vi "Assert Test SubVI.vi"(8 "error in (no error)":errorcluster) -> (0 "error out":errorcluster)   [LabVIEW 2009]
uses:
  classes/Assert/Assert.lvclass
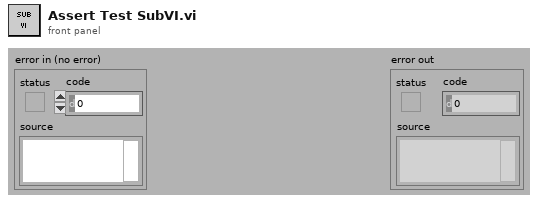
[diagram p1: front panel]
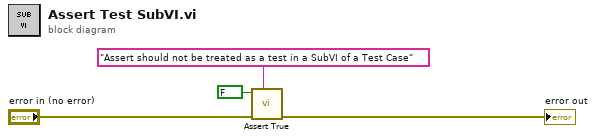
[diagram p0: block diagram]
diagram:
  n1 = call "Assert True.vi"("Label"="Assert should not be treated as a test in a SubVI of a Test Case", "error in (no error)"="error in (no error)", "True?"=FALSE) -> ("error out"=→"error out":errorcluster)  [unwired: 8 in]
